vi "Ref_Num_XYGraph_appearance.vi"(4 "Capacitance Results Temp Array":dbl[](array[numeric]), 5 "Test Voltages Results Temp Array":dbl[](array[numeric]), 8 "error in (no error)":errorcluster, 11 "XY Graph NEW":refnum<vi>) -> (0 "error out":errorcluster)   [LabVIEW 2020]
uses:
  Global 1.vi
panel:
  in  "Index Cluster":i32
  out "Array of DUT Cluster":cluster{"DUT (x)":dbl[], "DUT (y)":dbl[]}[](array[cluster])
  out "XY Graph Test":cluster{"DUT (x)":dbl[], "DUT (y)":dbl[]}[](graph)
  out "Display -> REFNUM : Test Voltages Results Temp Array":dbl[](array[numeric])
  out "Display -> REFNUM : Capacitance Results Temp Array":dbl[](array[numeric])
  in  "Array Size":i32
  out "Display -> GLOBAL VARIABLE : Array size(s)":i32
  # "To design algorithm for making the XY graph colorful"
  # "Index 0"
  # "Index 1"
  # "Index 2"
  # "TESTING in SUB VI"
  # "Capacitance in pF"
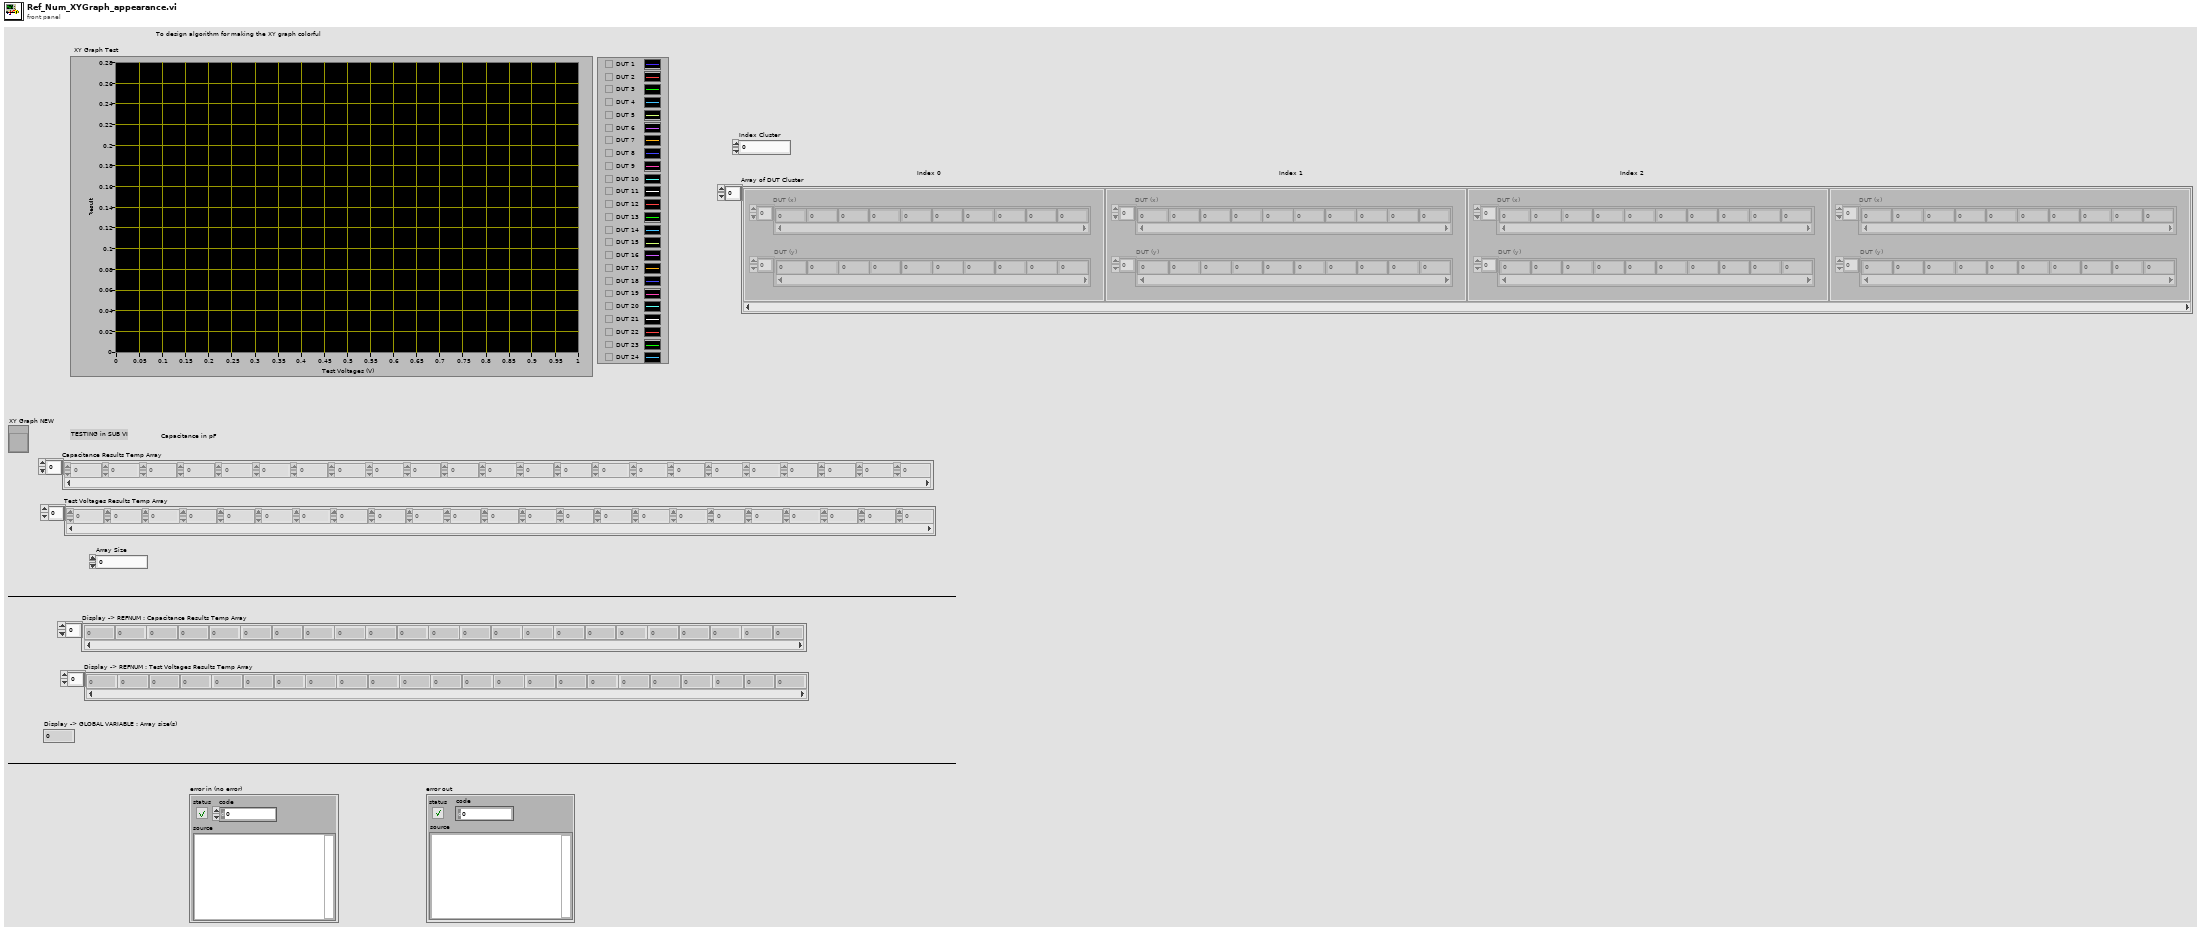
[diagram p1: front panel]
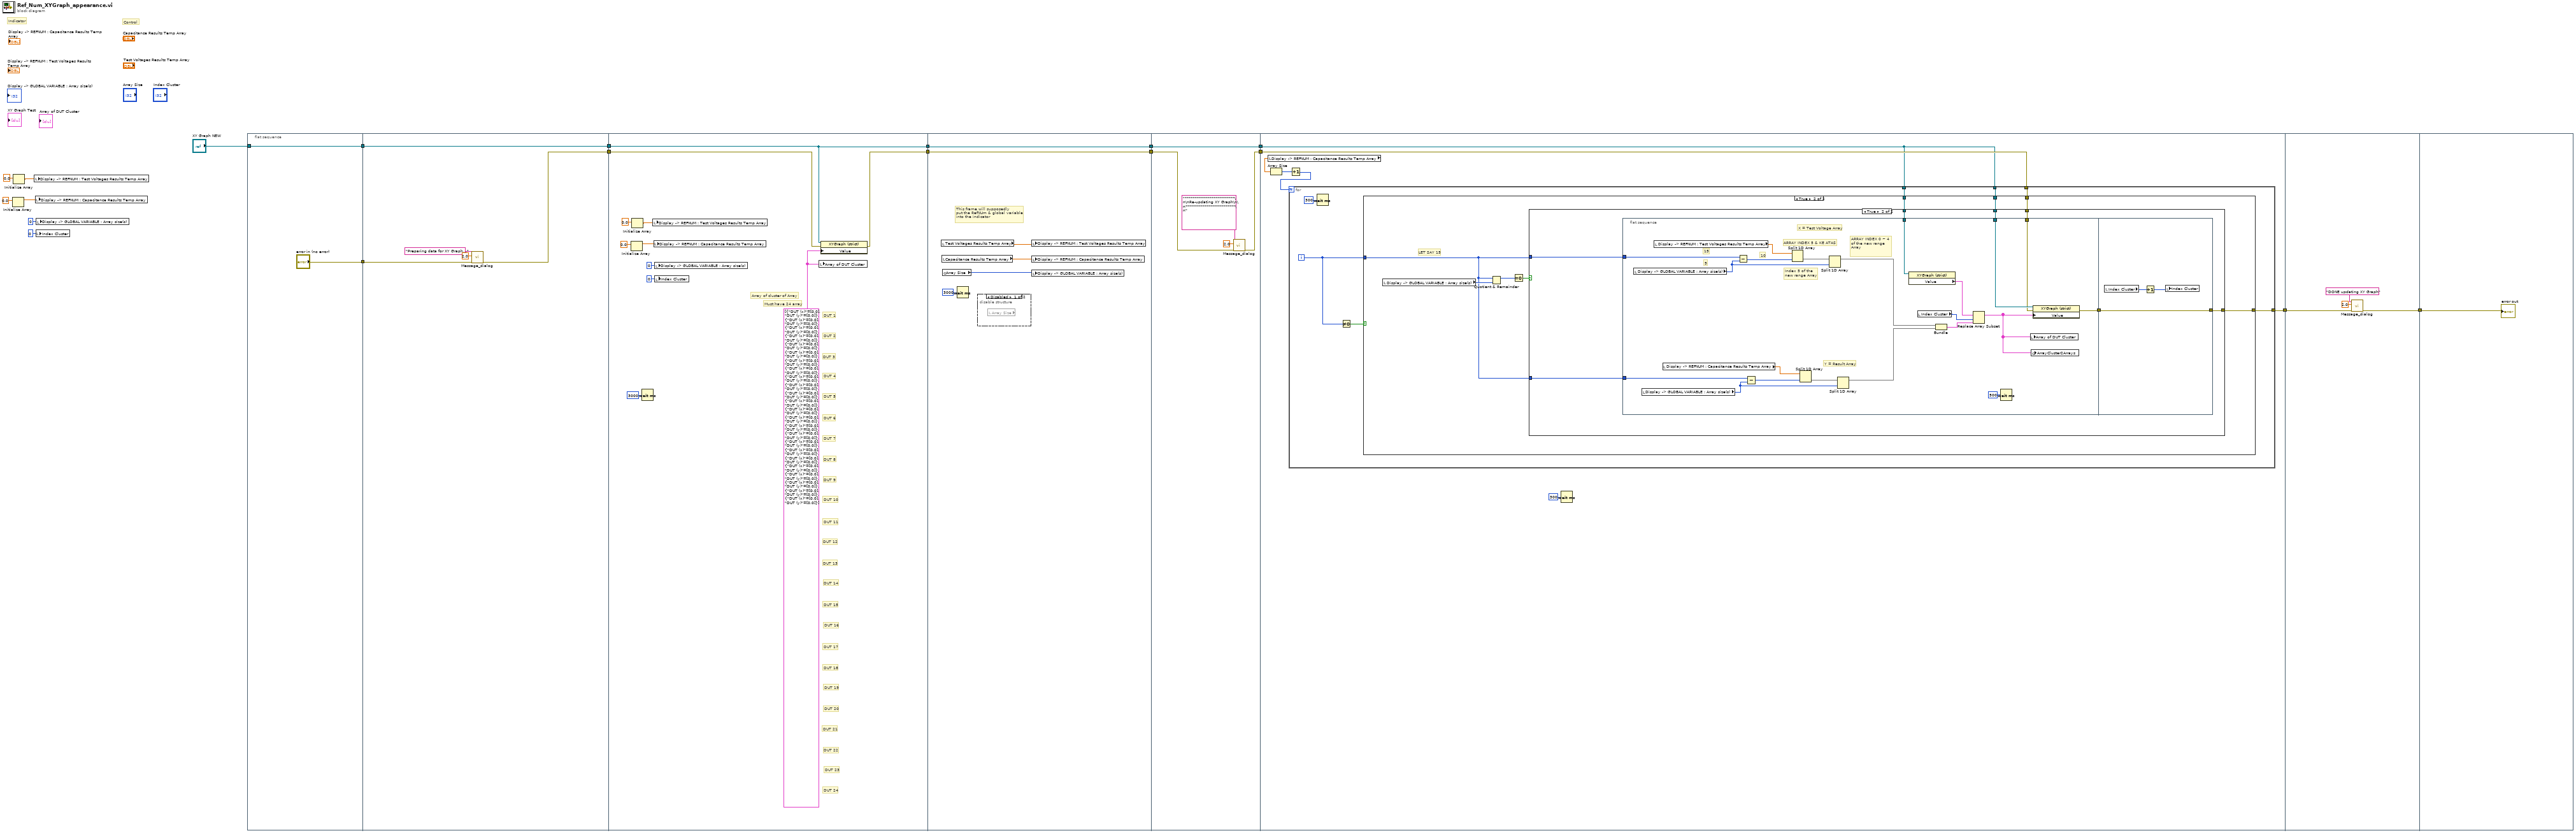
[diagram p0: block diagram]
diagram:
  # "Indicator"
  # "Control"
  n1 = Initialize Array(0.0 ("element")) -> (w4:dbl[])  [unwired: 1 in]
  n2 = Initialize Array(0.0 ("element")) -> (w3:dbl[])  [unwired: 1 in]
  n3 = local write "Display -> REFNUM : Test Voltages Results Temp Array"(w3) -> ()
  n4 = local write "Display -> REFNUM : Capacitance Results Temp Array"(w4) -> ()
  n5 = local write "Index Cluster"(0 ("Index Cluster")) -> ()
  n6 = local write "Display -> GLOBAL VARIABLE : Array size(s)"(0 ("Display -> GLOBAL VARIABLE : Array size(s)")) -> ()
  n7 = flat-sequence {
    tunnel: "XY Graph NEW" -> [w21]
    tunnel: [w21] -> w9
    tunnel: ["error in (no error)"] -> w8
    tunnel: [w26] -> w16
    tunnel: [w22] -> w11
    tunnel: w9 -> [w26]
    tunnel: w8 -> [w23]
    tunnel: [w31] -> w17
    tunnel: w16 -> [w31]
    tunnel: [w29] -> w13
    tunnel: w11 -> [w30]
    tunnel: [w40] -> w18
    tunnel: w17 -> [w40]
    tunnel: [w39] -> w14
    tunnel: w13 -> [w39]
    tunnel: [w48] -> w19
    tunnel: w18 -> [w48]
    tunnel: [w44] -> w15
    tunnel: w14 -> [w45]
    tunnel: w19 -> [w51]
    tunnel: w15 -> [w53]
    tunnel: [w52] -> w12
    tunnel: w12 -> [w105]
    tunnel: [w104] -> w10
    tunnel: w10 -> [w108]
    frame #0 {
    }
    frame #1 {
      n8 = call "Message_dialog.vi"("error in (no error)"=w23, "set delay"=2.0, "String"="Preparing data for XY Graph...") -> ("error out"=w22:errorcluster)  [unwired: 8 in]
    }
    frame #2 {
      w28 = cluster{"DUT (x)":dbl[], "DUT (y)":dbl[]}[] [{"DUT (x)"=[0.0], "DUT (y)"=[0.0]}, {"DUT (x)"=[0.0], "DUT (y)"=[0.0]}, {"DUT (x)"=[0.0], "DUT (y)"=[0.0]}, {"DUT (x)"=[0.0], "DUT (y)"=[0.0]}, {"DUT (x)"=[0.0], "DUT (y)"=[0.0]}, {"DUT (x)"=[0.0], "DUT (y)"=[0.0]}, {"DUT (x)"=[0.0], "DUT (y)"=[0.0]}, {"DUT (x)"=[0.0], "DUT (y)"=[0.0]}, {"DUT (x)"=[0.0], "DUT (y)"=[0.0]}, {"DUT (x)"=[0.0], "DUT (y)"=[0.0]}, {"DUT (x)"=[0.0], "DUT (y)"=[0.0]}, {"DUT (x)"=[0.0], "DUT (y)"=[0.0]}, {"DUT (x)"=[0.0], "DUT (y)"=[0.0]}, {"DUT (x)"=[0.0], "DUT (y)"=[0.0]}, {"DUT (x)"=[0.0], "DUT (y)"=[0.0]}, {"DUT (x)"=[0.0], "DUT (y)"=[0.0]}, {"DUT (x)"=[0.0], "DUT (y)"=[0.0]}, {"DUT (x)"=[0.0], "DUT (y)"=[0.0]}, {"DUT (x)"=[0.0], "DUT (y)"=[0.0]}, {"DUT (x)"=[0.0], "DUT (y)"=[0.0]}, {"DUT (x)"=[0.0], "DUT (y)"=[0.0]}, {"DUT (x)"=[0.0], "DUT (y)"=[0.0]}, {"DUT (x)"=[0.0], "DUT (y)"=[0.0]}, {"DUT (x)"=[0.0], "DUT (y)"=[0.0]}] ("Array of DUT Cluster")
      # "DUT 24"
      # "DUT 23"
      # "DUT 22"
      # "DUT 21"
      # "DUT 20"
      # "DUT 19"
      # "DUT 18"
      # "DUT 17"
      # "DUT 16"
      # "DUT 15"
      # "DUT 14"
      # "DUT 13"
      # "DUT 12"
      # "DUT 11"
      # "DUT 10"
      # "DUT 9"
      # "DUT 8"
      # "DUT 7"
      # "DUT 6"
      # "DUT 5"
      # "DUT 4"
      # "DUT 3"
      # "DUT 2"
      # "DUT 1"
      # "Array of cluster of Array"
      # "Must have 24 array"
      n9 = Initialize Array(0.0 ("element")) -> (w33:dbl[])  [unwired: 1 in]
      n10 = Initialize Array(0.0 ("element")) -> (w34:dbl[])  [unwired: 1 in]
      n11 = Wait (ms)(milliseconds to wait=u32 3000) -> ()  [unwired: 1 out]
      n12 = local write "Display -> REFNUM : Test Voltages Results Temp Array"(w34) -> ()
      n13 = local write "Display -> REFNUM : Capacitance Results Temp Array"(w33) -> ()
      n14 = local write "Display -> GLOBAL VARIABLE : Array size(s)"(0 ("Display -> GLOBAL VARIABLE : Array size(s)")) -> ()
      n15 = local write "Index Cluster"(0 ("Index Cluster")) -> ()
      n16 = local write "Array of DUT Cluster"(w28) -> ()
      n17 = property class="XYGraph (strict)"(reference=w31, error in=w30, "Value"=w28) -> (error out=w29:errorcluster)  [unwired: 1 out]
    }
    frame #3 {
      # "This frame will supposedly \nput the RefNUm & global variable\ninto the indicator"
      n18 = local read "Test Voltages Results Temp Array"() -> (w43:dbl[])
      n19 = local read "Capacitance Results Temp Array"() -> (w42:dbl[])
      n20 = global read "Global 1.vi" "Array Size"() -> (w38:i32)
      n21 = Wait (ms)(milliseconds to wait=u32 3000) -> ()  [unwired: 1 out]
      n22 = disable-structure shown="Disabled" {
        frame Disabled {
          n23 = local read "Array Size"() -> ()  [unwired: 1 out]
        }
        frame Enabled {
        }
      }
      n24 = local write "Display -> REFNUM : Test Voltages Results Temp Array"(w43) -> ()
      n25 = local write "Display -> REFNUM : Capacitance Results Temp Array"(w42) -> ()
      n26 = local write "Display -> GLOBAL VARIABLE : Array size(s)"(w38) -> ()
    }
    frame #4 {
      n27 = call "Message_dialog.vi"("error in (no error)"=w45, "set delay"=2.0, "String"="**************************\n\nRe-updating XY Graph\n\n**************************\n") -> ("error out"=w44:errorcluster)  [unwired: 8 in]
    }
    frame #5 {
      n28 = local read "Display -> REFNUM : Capacitance Results Temp Array"() -> (w55:dbl[])
      n29 = Array Size(array=w55) -> (size(s)=w50:i32)
      n30 = Increment(x=w50) -> (x+1=w49:i32)
      n31 = for {
        N: w49 -> [_]
        tunnel: w51 -> [w62]
        tunnel: w53 -> [w60]
        tunnel: [w59] -> w52
        tunnel: w51 -> [w58]
        i -> [w57]
        n32 = Wait (ms)(milliseconds to wait=u32 300) -> ()  [unwired: 1 out]
        n33 = Not Equal To 0?(x=w57) -> (x != 0?=w56:bool)
        n34 = case shown="True" w56 {
          tunnel: w62 -> [_ w68]
          tunnel: w60 -> [w63 w67]
          tunnel: [w63 w66] -> w59
          tunnel: w58 -> [_ w65]
          tunnel: w57 -> [_ w64]
          frame False {
          }
          frame True {
            # "LET SAY 15"
            n35 = local read "Display -> GLOBAL VARIABLE : Array size(s)"() -> (w71:i32)
            n36 = Quotient & Remainder(x=w64, y=w71) -> (x-y*floor(x/y)=w70:i32)  [unwired: 1 out]
            n37 = Equal To 0?(x=w70) -> (x = 0?=w69:bool)
            n38 = case shown="True" w69 {
              tunnel: w64 -> [_ w79]
              tunnel: w64 -> [_ w78]
              tunnel: w68 -> [_ w77]
              tunnel: w67 -> [w72 w76]
              tunnel: [w72 w75] -> w66
              tunnel: w65 -> [_ w74]
              frame False {
              }
              frame True {
                n39 = flat-sequence {
                  tunnel: w79 -> [w83]
                  tunnel: w78 -> [w84]
                  tunnel: w77 -> [w96]
                  tunnel: w76 -> [w95]
                  tunnel: w74 -> [w91]
                  tunnel: [w94] -> w73
                  tunnel: [w103] -> w75
                  tunnel: w73 -> [w103]
                  frame #0 {
                    # "Index 5 of the\nnew range Array"
                    # "ARRAY INDEX 0 ~ 4\nof the new range Array"
                    # "ARRAY INDEX 5 & KE ATAS"
                    # "10"
                    # "5"
                    # "15"
                    # "Y = Result Array"
                    # "X = Test Voltage Array"
                    n40 = local read "Display -> GLOBAL VARIABLE : Array size(s)"() -> (w82:i32)
                    n41 = local read "Display -> GLOBAL VARIABLE : Array size(s)"() -> (w81:i32)
                    n42 = local read "Display -> REFNUM : Test Voltages Results Temp Array"() -> (w99:dbl[])
                    n43 = local read "Display -> REFNUM : Capacitance Results Temp Array"() -> (w97:dbl[])
                    n44 = Subtract(x=w83, y=w82) -> (x-y=w87:i32)
                    n45 = Subtract(x=w84, y=w81) -> (x-y=w85:i32)
                    n46 = Split 1D Array(array=w99, index=w87) -> (second subarray=w100:dbl[])  [unwired: 1 out]
                    n47 = Split 1D Array(array=w97, index=w85) -> (second subarray=w98:dbl[])  [unwired: 1 out]
                    n48 = Split 1D Array(array=w100, index=w82) -> (first subarray=w93:dbl[])  [unwired: 1 out]
                    n49 = Split 1D Array(array=w98, index=w81) -> (first subarray=w92:dbl[])  [unwired: 1 out]
                    n50 = property class="XYGraph (strict)"(reference=w91) -> ("Value"=w90:cluster{"DUT (x)":dbl[], "DUT (y)":dbl[]}[])  [unwired: 1 in, 2 out]
                    n51 = local read "Index Cluster"() -> (w88:i32)
                    n52 = Bundle(w93, w92) -> (w89:cluster{dbl[], dbl[]})  [unwired: 1 in]
                    n53 = Replace Array Subset(array=w90, new element=w89, index=w88) -> (w80:cluster{"DUT (x)":dbl[], "DUT (y)":dbl[]}[])
                    n54 = Wait (ms)(milliseconds to wait=u32 500) -> ()  [unwired: 1 out]
                    n55 = local write "Array of DUT Cluster"(w80) -> ()
                    n56 = global write "Global 1.vi" "ArrayCluster2Arrays"(w80) -> ()
                    n57 = property class="XYGraph (strict)"(reference=w96, error in=w95, "Value"=w80) -> (error out=w94:errorcluster)  [unwired: 1 out]
                  }
                  frame #1 {
                    n58 = local read "Index Cluster"() -> (w102:i32)
                    n59 = Increment(x=w102) -> (x+1=w101:i32)
                    n60 = local write "Index Cluster"(w101) -> ()
                  }
                }
              }
            }
          }
        }
      }
      n61 = Wait (ms)(milliseconds to wait=u32 300) -> ()  [unwired: 1 out]
    }
    frame #6 {
      n62 = call "Message_dialog.vi"("error in (no error)"=w105, "set delay"=2.0, "String"="DONE updating XY Graph") -> ("error out"=w104:errorcluster)  [unwired: 8 in]
    }
    frame #7 {
      "error out" <- w108
    }
  }
